vi "read_attributes.vi"(8 "error in (no error)":errorcluster, 11 "LogisticRegressionCV in":refnum<class "LogisticRegressionCV.lvclass">) -> (0 "error out":errorcluster, 2 "attributes":T1, 3 "LogisticRegressionCV out":refnum<class "LogisticRegressionCV.lvclass">)   [LabVIEW 2020, in "LogisticRegressionCV.lvclass"]
uses:
  LogisticRegressionCV.lvclass
  Controls/logistic_regression_cv_attributes.ctl
  LogisticRegressionCV.lvclass/LogisticRegressionCV.ctl
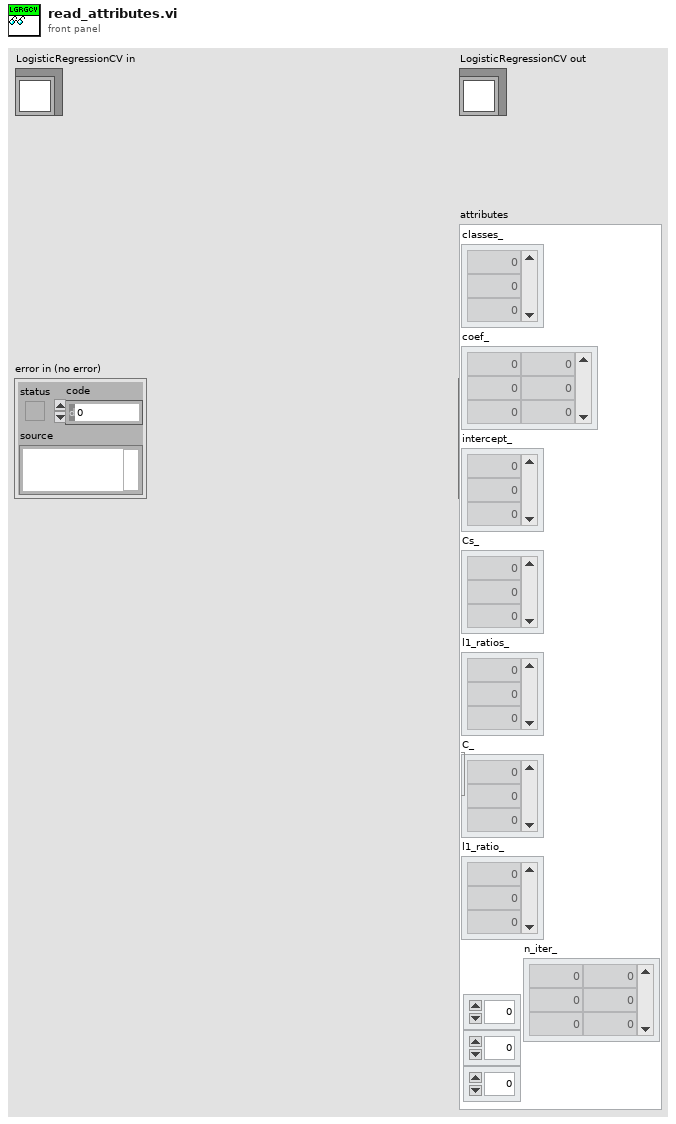
[diagram p1: front panel]
types:
  T1 = typedef "logistic_regression_cv_attributes.ctl" = cluster{"classes_":dbl[], "coef_":dbl[][], "intercept_":dbl[], "Cs_":dbl[], "l1_ratios_":dbl[], "C_":dbl[], "l1_ratio_":dbl[], "n_iter_":dbl[][][][]}
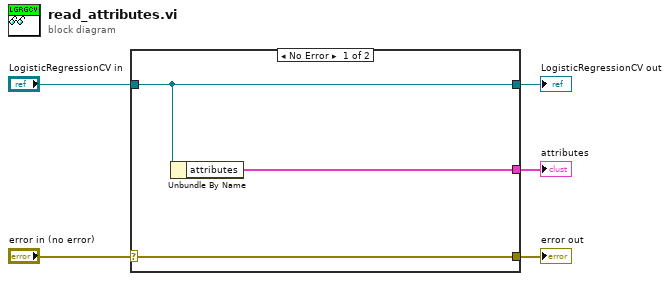
[diagram p0: block diagram]
diagram:
  n1 = case shown="No Error" "error in (no error)" {
    selector: "error in (no error)" -> [w8 w9]
    tunnel: [w8 w9] -> w4
    tunnel: [w7 w10] -> w2
    tunnel: "LogisticRegressionCV in" -> [w7 w10]
    tunnel: [w6 _] -> w1
    frame No Error {
      n2 = Unbundle By Name(w7) -> ("attributes"=w6:T1)
    }
    frame Error {
    }
  }
  "error out" <- w4
  "LogisticRegressionCV out" <- w2
  "attributes" <- w1
